vi "FileSync.Get Status.vi"(8 "error in (no error)":errorcluster, 11 "File.Sync in":refnum<class "File.Sync.lvclass">) -> (0 "error out":errorcluster, 1 "Event Log":T2[](array[typedef]), 2 "Sync Items":T1[](array[typedef]), 3 "File.Sync out":refnum<class "File.Sync.lvclass">)   [LabVIEW 2024, in "KATE_Lib.lvlib" / "File Utils.lvlib" / "File.Sync.lvclass"]
uses:
  File.Sync.lvclass
  File.Sync Item Log Record.ctl
  File.Sync Item Record.ctl
  File.Sync.lvclass/File.Sync.ctl
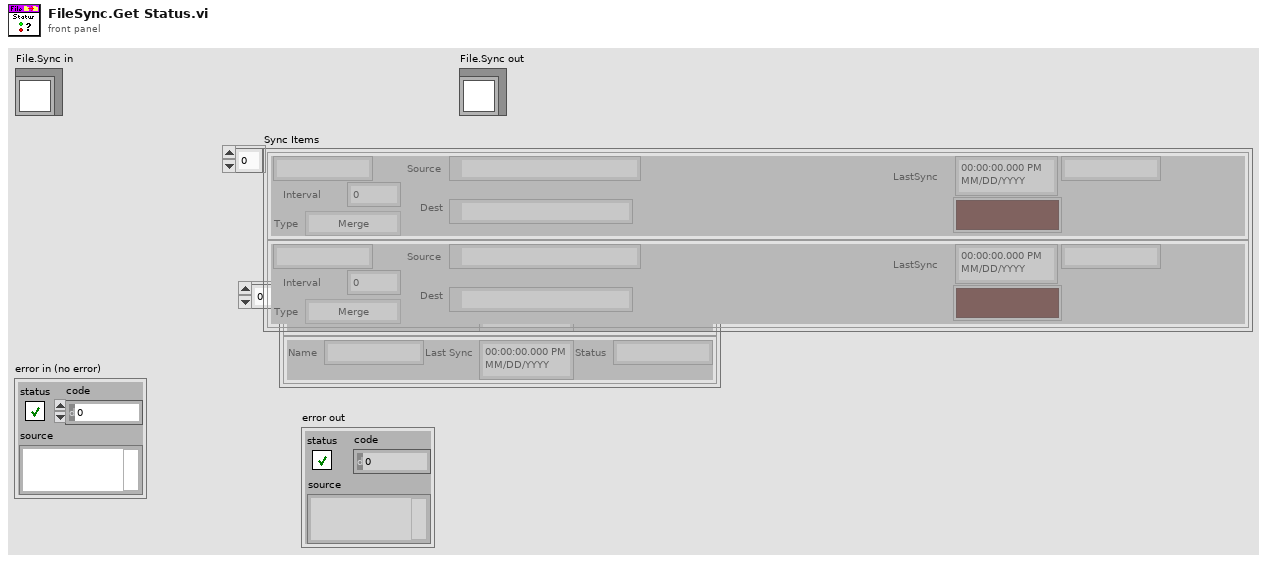
[diagram p1: front panel]
types:
  T1 = typedef "KATE_Lib.lvlib/File Utils.lvlib/File.Sync.lvclass/File.Sync Item Record.ctl" = cluster{"Name":string, "Interval":dbl, "Source":path, "Dest":path, "LastSync":timestamp, "Status":string, "Error":bool, "Type":enum16{"Merge", "Match"}}
  T2 = typedef "KATE_Lib.lvlib/File Utils.lvlib/File.Sync.lvclass/File.Sync Item Log Record.ctl" = cluster{"Name":string, "Last Sync":timestamp, "Status":string}
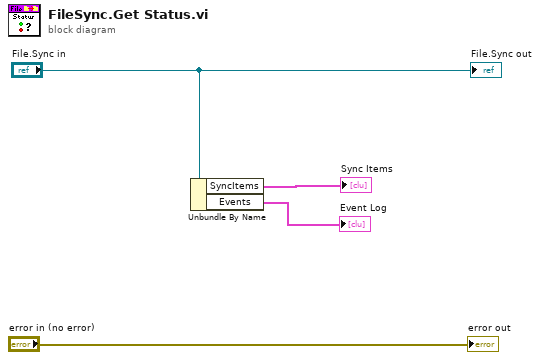
[diagram p0: block diagram]
diagram:
  n1 = Unbundle By Name("File.Sync in") -> ("SyncItems"=→"Sync Items":T1[], "Events"=→"Event Log":T2[])
  "error out" <- "error in (no error)"
  "File.Sync out" <- "File.Sync in"
